vi "UI Flow Rate of Wash Tank.vi"(8 "error in":errorcluster) -> (0 "error out":errorcluster)   [LabVIEW 2019, in "Test.lvlib"]
uses:
  Test.lvlib
  Fluidic Process/SubVI/Fluidic Para.ctl
  <vilib>/Utility/file.llb/Read Delimited Spreadsheet (string).vi
  Controller/Controller.lvlib
  Queues/Queues.lvlib
  Fluidic Process/Fluidic Process.lvlib
panel:
  in  "Stop Process":bool
  out "Remaining Time(s)":dbl
  out "Total Process":string
  out "Current Process":string
  out "Gauge":dbl(knob)=1.2869315802184793e-48 scale=0.0..100.0
  in  "Wash Load R":bool
  in  "Wash Load L":bool
  in  "Back":bool
  # "/"
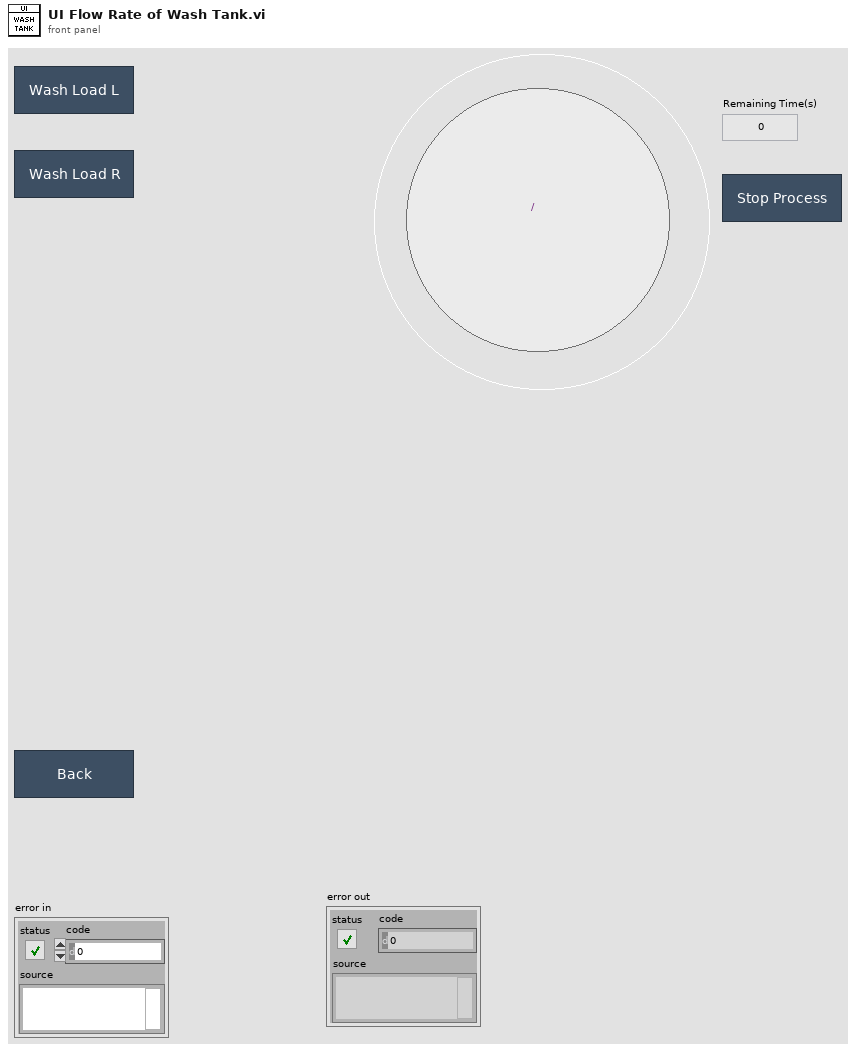
[diagram p1: front panel]
types:
  T1 = enum8{"Enabled", "Disabled", "Disabled and Grayed Out"}
  T2 = typedef "Fluidic Process.lvlib/Fluidic Para.ctl" = cluster{"Read Force Sensor":i32, "Read Regulator":i32, "Read Force Sensor?":bool, "Read Regulator?":bool, "Read Syringe Pump":i32, "Read Syringe Pump?":bool}
  T3 = typedef "Fluidic Process.lvlib/SEQ Data.ctl" = cluster{"Fluidic Process Done?":bool, "Current Process":i32, "Remaining Time":dbl, "Total Process":i32, "Air Sealing":bool, "Force Condition":bool}
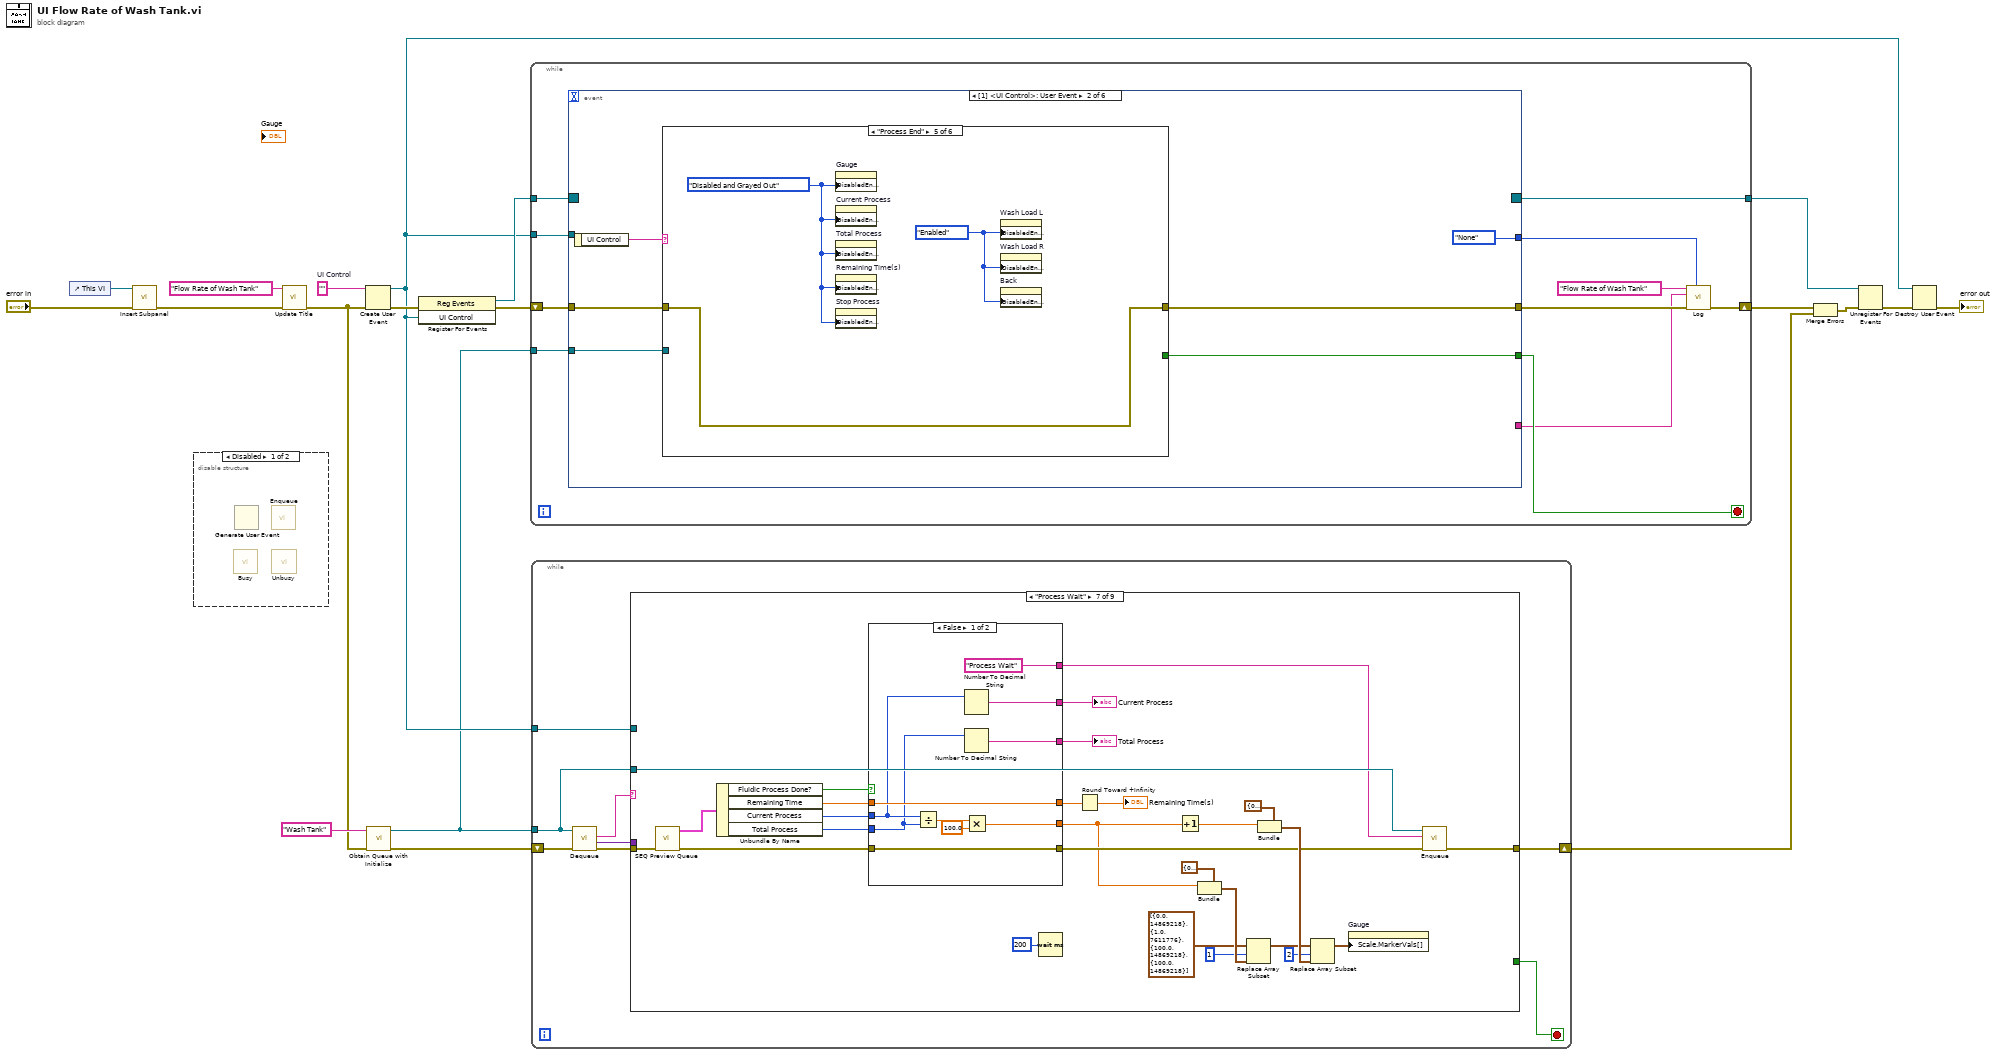
[diagram p0: block diagram]
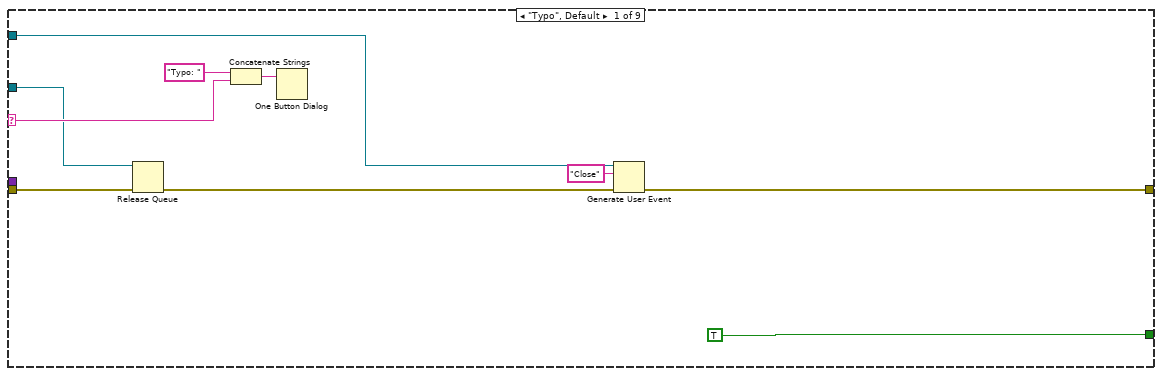
[diagram p3: hidden frame]
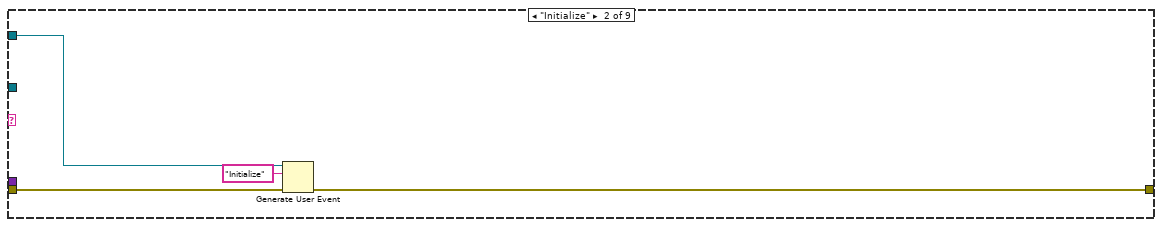
[diagram p4: hidden frame]
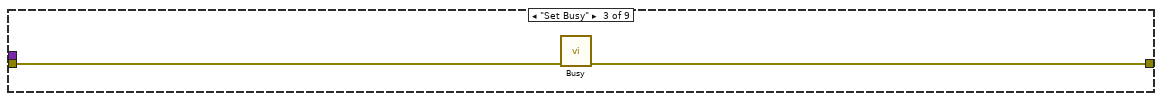
[diagram p5: hidden frame]
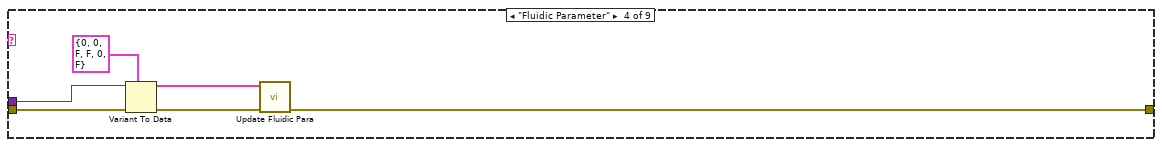
[diagram p6: hidden frame]
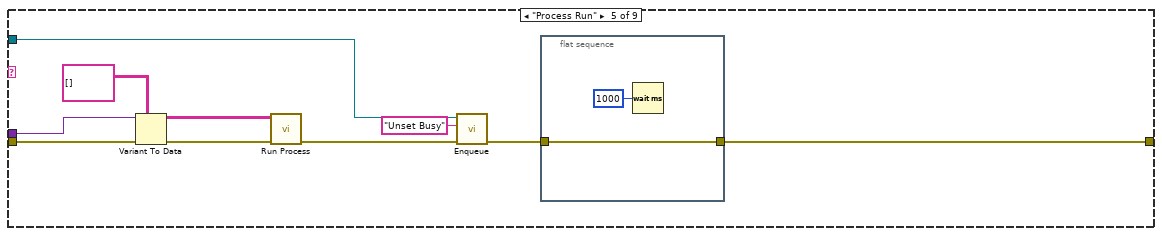
[diagram p7: hidden frame]
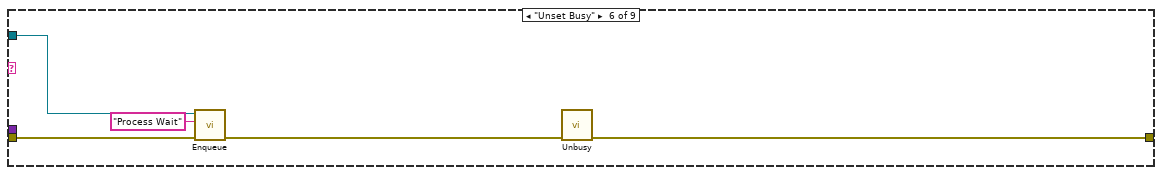
[diagram p8: hidden frame]
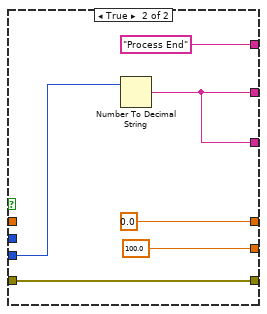
[diagram p9: hidden frame]
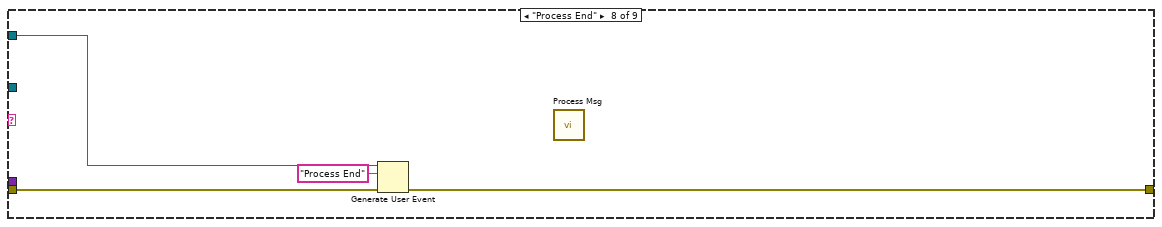
[diagram p10: hidden frame]
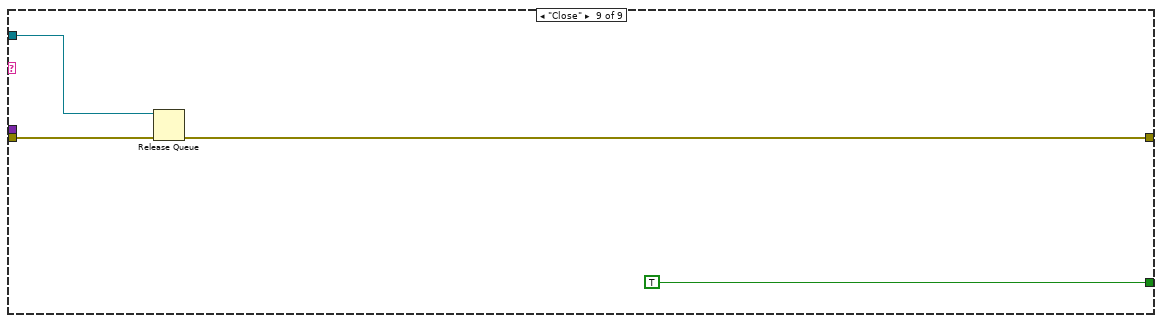
[diagram p11: hidden frame]
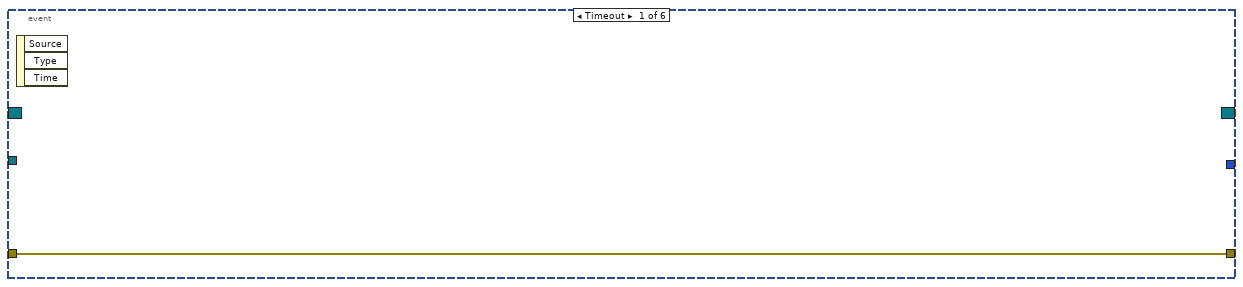
[diagram p12: hidden frame]
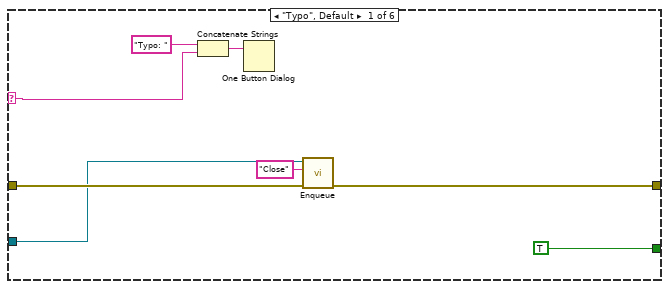
[diagram p13: hidden frame]
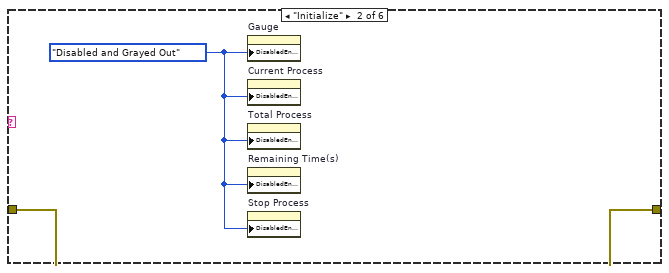
[diagram p14: hidden frame]
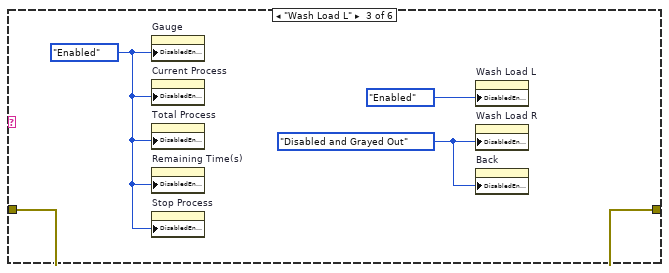
[diagram p15: hidden frame]
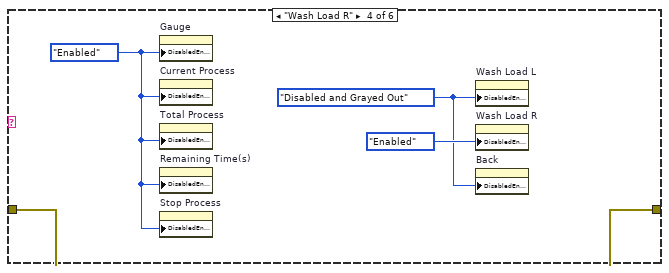
[diagram p16: hidden frame]
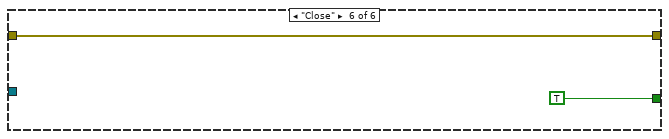
[diagram p17: hidden frame]
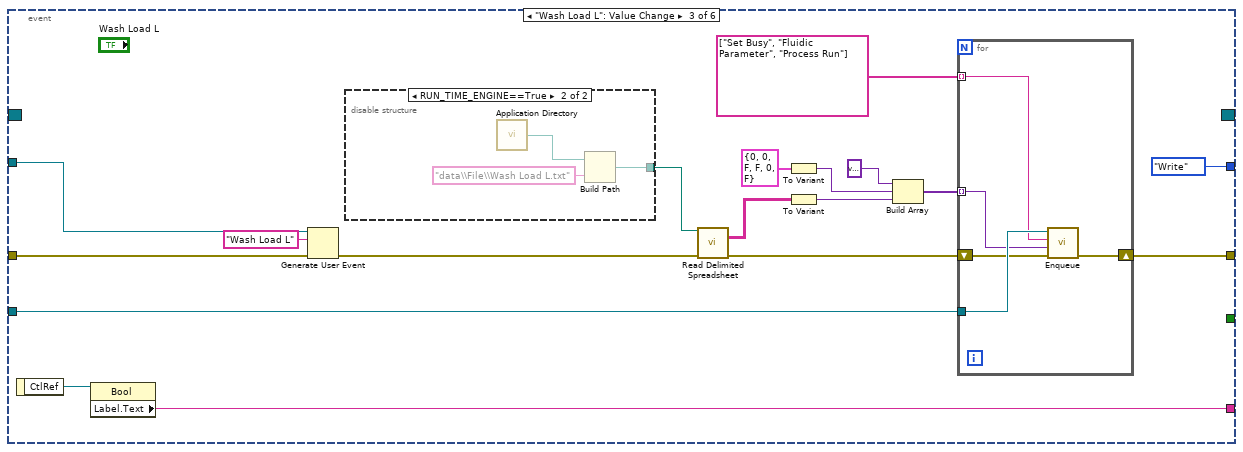
[diagram p18: hidden frame]
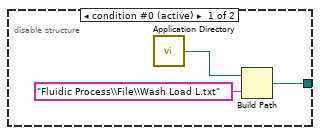
[diagram p19: hidden frame]
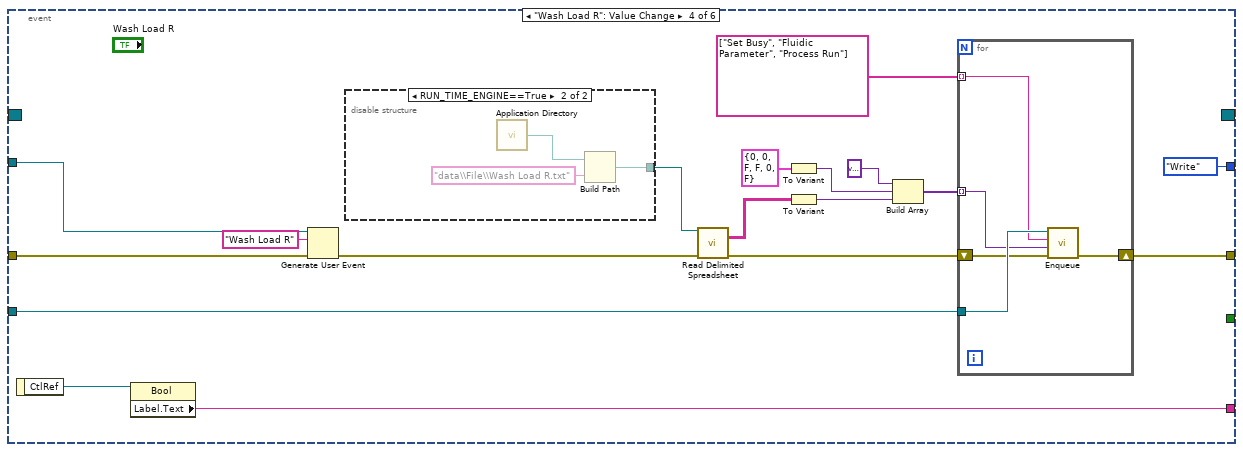
[diagram p20: hidden frame]
diagram:
  w9 = ""  # UI Control
  n1 = control-ref of="This VI"() -> (w8:refnum<vi>)
  n2 = call "Insert Subpanel.vi"("Error In"="error in", "VI Refnum"=w8) -> ("Error Out"=w3:errorcluster)  [unwired: 9 in]
  n3 = disable-structure shown="Disabled" {
    frame Disabled {
      n4 = call "Busy.vi"() -> ()  [unwired: 11 in, 1 out]
      n5 = Generate User Event() -> ()  [unwired: 4 in, 2 out]
      n6 = call "Enqueue.vi"() -> ()  [unwired: 10 in, 2 out]
      n7 = call "Unbusy.vi"() -> ()  [unwired: 11 in, 1 out]
    }
    frame Enabled {
    }
  }
  n8 = call "Update Title.vi"("Error In"=w3, "Title"="Flow Rate of Wash Tank") -> ("Error Out"=w2:errorcluster)  [unwired: 9 in]
  n9 = Create User Event(user event datatype=w9, error in=w2) -> (user event=w7:refnum<user-event>, error out=w18:errorcluster)
  n10 = call "Obtain Queue with Initialize.vi"("Error In"=w2, "Queue Name"="Wash Tank") -> ("Error Out"=w4:errorcluster, "Queue out"=w5:refnum<queue>)  [unwired: 8 in]
  n11 = register-events(error in=w18, w7) -> (reference out=w16:refnum<event-registration>, error out=w17:errorcluster)  [unwired: 1 in]
  n12 = while {
    tunnel: w16 -> [w28]
    tunnel: w5 -> [w27]
    shift-right: [w23] -> w14
    shift-left: w17 -> [w30]
    tunnel: [w26] -> w12
    tunnel: w7 -> [w25]
    stop <- w29 stop-if-true
    n13 = event shown="[1] <UI Control>: User Event" {
      selector: w28 -> [_ _ _ _ _ _]
      dyn-events: [_ _ _ _ _ _] -> w26
      timeout: _ -> [_ _ _ _ _ _]
      tunnel: w30 -> [w31 w37 w67 w96 w123 w127]
      tunnel: [_ w33 _ _ _ TRUE] -> w29
      tunnel: w27 -> [_ w35 w78 w107 _ w129]
      tunnel: [w31 w34 w74 w103 w122 w130] -> w24
      tunnel: w25 -> [_ _ w65 w94 _ _]
      tunnel: [_ enum16{"None", "Write"}."None" ("Action") enum16{"None", "Write"}."Write" ("Action") enum16{"None", "Write"}."Write" ("Action") enum16{"None", "Write"}."Write" ("Action") enum16{"None", "Write"}."Write" ("Action")] -> w21
      tunnel: [_ _ w61 w90 w120 w125] -> w20
      event Timeout {
        n14 = event-data() -> ()  [unwired: 1 in, 3 out]
      }
      event User Event {
        n15 = event-data() -> ("UI Control"=w36:string)  [unwired: 1 in]
        n16 = case shown="\"Process End\"" w36 {
          selector: w36 -> [w40 _ _ _ _ _]
          tunnel: w37 -> [w45 w47 w51 w55 w58 w60]
          tunnel: w35 -> [w44 _ _ _ _ _]
          tunnel: [w39 w47 w51 w55 w58 w60] -> w34
          tunnel: [TRUE _ _ _ _ TRUE] -> w33
          frame "Typo", Default {
            n17 = Concatenate Strings("Typo: " ("string"), w40) -> (w41:string)
            n18 = One Button Dialog(message=w41) -> ()  [unwired: 1 in, 1 out]
            n19 = call "Enqueue.vi"("Error In"=w45, "State"="Close", "Queue in"=w44) -> ("Error Out"=w39:errorcluster)  [unwired: 7 in, 1 out]
          }
          frame "Initialize" {
            w46 = T1."Disabled and Grayed Out" ("Disabled")
            n20 = property on="Gauge" class="Knob (strict)"("DisabledEnum"=w46) -> ()  [unwired: 2 in, 2 out]
            n21 = property on="Current Process" class="Str"("DisabledEnum"=w46) -> ()  [unwired: 2 in, 2 out]
            n22 = property on="Total Process" class="Str"("DisabledEnum"=w46) -> ()  [unwired: 2 in, 2 out]
            n23 = property on="Remaining Time(s)" class="DigNum (strict)"("DisabledEnum"=w46) -> ()  [unwired: 2 in, 2 out]
            n24 = property on="Stop Process" class="Bool"("DisabledEnum"=w46) -> ()  [unwired: 2 in, 2 out]
          }
          frame "Wash Load L" {
            w49 = T1."Enabled" ("Disabled")
            w48 = T1."Disabled and Grayed Out" ("Disabled")
            n25 = property on="Gauge" class="Knob (strict)"("DisabledEnum"=w49) -> ()  [unwired: 2 in, 2 out]
            n26 = property on="Current Process" class="Str"("DisabledEnum"=w49) -> ()  [unwired: 2 in, 2 out]
            n27 = property on="Total Process" class="Str"("DisabledEnum"=w49) -> ()  [unwired: 2 in, 2 out]
            n28 = property on="Remaining Time(s)" class="DigNum (strict)"("DisabledEnum"=w49) -> ()  [unwired: 2 in, 2 out]
            n29 = property on="Stop Process" class="Bool"("DisabledEnum"=w49) -> ()  [unwired: 2 in, 2 out]
            n30 = property on="Wash Load L" class="Bool"("DisabledEnum"=T1."Enabled" ("Disabled")) -> ()  [unwired: 2 in, 2 out]
            n31 = property on="Wash Load R" class="Bool"("DisabledEnum"=w48) -> ()  [unwired: 2 in, 2 out]
            n32 = property on="Back" class="Bool"("DisabledEnum"=w48) -> ()  [unwired: 2 in, 2 out]
          }
          frame "Wash Load R" {
            w53 = T1."Enabled" ("Disabled")
            w52 = T1."Disabled and Grayed Out" ("Disabled")
            n33 = property on="Gauge" class="Knob (strict)"("DisabledEnum"=w53) -> ()  [unwired: 2 in, 2 out]
            n34 = property on="Current Process" class="Str"("DisabledEnum"=w53) -> ()  [unwired: 2 in, 2 out]
            n35 = property on="Total Process" class="Str"("DisabledEnum"=w53) -> ()  [unwired: 2 in, 2 out]
            n36 = property on="Remaining Time(s)" class="DigNum (strict)"("DisabledEnum"=w53) -> ()  [unwired: 2 in, 2 out]
            n37 = property on="Stop Process" class="Bool"("DisabledEnum"=w53) -> ()  [unwired: 2 in, 2 out]
            n38 = property on="Wash Load L" class="Bool"("DisabledEnum"=w52) -> ()  [unwired: 2 in, 2 out]
            n39 = property on="Wash Load R" class="Bool"("DisabledEnum"=T1."Enabled" ("Disabled")) -> ()  [unwired: 2 in, 2 out]
            n40 = property on="Back" class="Bool"("DisabledEnum"=w52) -> ()  [unwired: 2 in, 2 out]
          }
          frame "Process End" {
            w57 = T1."Disabled and Grayed Out" ("Disabled")
            w56 = T1."Enabled" ("Disabled")
            n41 = property on="Gauge" class="Knob (strict)"("DisabledEnum"=w57) -> ()  [unwired: 2 in, 2 out]
            n42 = property on="Current Process" class="Str"("DisabledEnum"=w57) -> ()  [unwired: 2 in, 2 out]
            n43 = property on="Total Process" class="Str"("DisabledEnum"=w57) -> ()  [unwired: 2 in, 2 out]
            n44 = property on="Remaining Time(s)" class="DigNum (strict)"("DisabledEnum"=w57) -> ()  [unwired: 2 in, 2 out]
            n45 = property on="Stop Process" class="Bool"("DisabledEnum"=w57) -> ()  [unwired: 2 in, 2 out]
            n46 = property on="Wash Load L" class="Bool"("DisabledEnum"=w56) -> ()  [unwired: 2 in, 2 out]
            n47 = property on="Wash Load R" class="Bool"("DisabledEnum"=w56) -> ()  [unwired: 2 in, 2 out]
            n48 = property on="Back" class="Bool"("DisabledEnum"=w56) -> ()  [unwired: 2 in, 2 out]
          }
          frame "Close" {
          }
        }
      }
      event "Wash Load L": Value Change {
        n49 = event-data() -> ("CtlRef"=w62:refnum<vi>)  [unwired: 1 in]
        n50 = property class="Bool"(reference=w62) -> ("Label.Text"=w61:string)  [unwired: 1 in, 2 out]
        n51 = Generate User Event(user event=w65, event data cluster="Wash Load L" ("event data"), error in=w67) -> (error out=w66:errorcluster)  [unwired: 1 in, 1 out]
        n52 = disable-structure shown="RUN_TIME_ENGINE==True" {
          disable-tunnel: [w79 w82] -> w76
          frame condition #0 (active) {
            n53 = call <vilib>:"Application Directory.vi"() -> ("Application Directory"=w81:path)
            n54 = Build Path(base path=w81, name or relative path="Fluidic Process\\File\\Wash Load L.txt") -> (appended path=w79:path)
          }
          frame condition #1 {
            n55 = call <vilib>:"Application Directory.vi"() -> ("Application Directory"=w84:path)
            n56 = Build Path(base path=w84, name or relative path="data\\File\\Wash Load L.txt") -> (appended path=w82:path)
          }
        }
        n57 = call-poly <vilib>:"Read Delimited Spreadsheet.vi"("file path (dialog if empty)"=w76, "error in (no error)"=w66) -> ("all rows"=w75:string[][], "error out"=w77:errorcluster)  [unwired: 8 in, 4 out]
        n58 = To Variant(anything=T2 {"Read Force Sensor"=0, "Read Regulator"=0, "Read Force Sensor?"=FALSE, "Read Regulator?"=FALSE, "Read Syringe Pump"=0, "Read Syringe Pump?"=FALSE} ("Cluster")) -> (Variant=w70:variant)
        n59 = To Variant(anything=w75) -> (Variant=w72:variant)
        n60 = Build Array(variant, w70, w72) -> (w69:variant[])
        n61 = for {
          tunnel: w78 -> [w89]
          shift-right: [w87] -> w74
          shift-left: w77 -> [w88]
          tunnel: string[] ["Set Busy", "Fluidic Parameter", "Process Run"] -> [w86] mode=indexing
          tunnel: w69 -> [w85] mode=indexing
          n62 = call "Enqueue.vi"("Error In"=w88, "Data"=w85, "State"=w86, "Queue in"=w89) -> ("Error Out"=w87:errorcluster)  [unwired: 6 in, 1 out]
        }
      }
      event "Wash Load R": Value Change {
        n63 = event-data() -> ("CtlRef"=w91:refnum<vi>)  [unwired: 1 in]
        n64 = property class="Bool"(reference=w91) -> ("Label.Text"=w90:string)  [unwired: 1 in, 2 out]
        n65 = Generate User Event(user event=w94, event data cluster="Wash Load R" ("event data"), error in=w96) -> (error out=w95:errorcluster)  [unwired: 1 in, 1 out]
        n66 = disable-structure shown="RUN_TIME_ENGINE==True" {
          disable-tunnel: [w108 w111] -> w105
          frame condition #0 (active) {
            n67 = call <vilib>:"Application Directory.vi"() -> ("Application Directory"=w110:path)
            n68 = Build Path(base path=w110, name or relative path="Fluidic Process\\File\\Wash Load R.txt") -> (appended path=w108:path)
          }
          frame condition #1 {
            n69 = call <vilib>:"Application Directory.vi"() -> ("Application Directory"=w113:path)
            n70 = Build Path(base path=w113, name or relative path="data\\File\\Wash Load R.txt") -> (appended path=w111:path)
          }
        }
        n71 = call-poly <vilib>:"Read Delimited Spreadsheet.vi"("file path (dialog if empty)"=w105, "error in (no error)"=w95) -> ("all rows"=w104:string[][], "error out"=w106:errorcluster)  [unwired: 8 in, 4 out]
        n72 = To Variant(anything=T2 {"Read Force Sensor"=0, "Read Regulator"=0, "Read Force Sensor?"=FALSE, "Read Regulator?"=FALSE, "Read Syringe Pump"=0, "Read Syringe Pump?"=FALSE} ("Cluster")) -> (Variant=w99:variant)
        n73 = To Variant(anything=w104) -> (Variant=w101:variant)
        n74 = Build Array(variant, w99, w101) -> (w98:variant[])
        n75 = for {
          tunnel: w107 -> [w118]
          shift-right: [w116] -> w103
          shift-left: w106 -> [w117]
          tunnel: string[] ["Set Busy", "Fluidic Parameter", "Process Run"] -> [w115] mode=indexing
          tunnel: w98 -> [w114] mode=indexing
          n76 = call "Enqueue.vi"("Error In"=w117, "Data"=w114, "State"=w115, "Queue in"=w118) -> ("Error Out"=w116:errorcluster)  [unwired: 6 in, 1 out]
        }
      }
      event "Stop Process": Value Change {
        n77 = event-data() -> ("CtlRef"=w121:refnum<vi>)  [unwired: 1 in]
        n78 = property class="Bool"(reference=w121) -> ("Label.Text"=w120:string)  [unwired: 1 in, 2 out]
        n79 = call "Stop Process.vi"("Error In"=w123) -> ("Error Out"=w122:errorcluster)  [unwired: 10 in]
      }
      event "Back": Value Change {
        n80 = event-data() -> ("CtlRef"=w126:refnum<vi>)  [unwired: 1 in]
        n81 = property class="Bool"(reference=w126) -> ("Label.Text"=w125:string)  [unwired: 1 in, 2 out]
        n82 = call "Enqueue.vi"("Error In"=w127, "State"="Close", "Queue in"=w129) -> ("Error Out"=w130:errorcluster)  [unwired: 7 in, 1 out]
      }
    }
    n83 = call "Log.vi"("Action"=w21, "error in"=w24, "State"=w20, "Page Name"="Flow Rate of Wash Tank") -> ("error out"=w23:errorcluster)  [unwired: 7 in]
  }
  n84 = while {
    tunnel: w5 -> [w136]
    shift-right: [w134] -> w13
    shift-left: w4 -> [w139]
    tunnel: w7 -> [w133]
    stop <- w132 stop-if-true
    n85 = call "Dequeue.vi"("Error In"=w139, "Queue in"=w136) -> ("Error Out"=w135:errorcluster, "Data"=w137:variant, "State"=w138:string)  [unwired: 6 in, 1 out]
    n86 = case shown="\"Process Wait\"" w138 {
      selector: w138 -> [w147 _ _ _ _ _ _ _ _]
      tunnel: w137 -> [_ _ _ w160 w170 _ _ _ _]
      tunnel: w136 -> [w140 _ _ _ w165 w177 w183 _ w227]
      tunnel: w135 -> [w142 w153 w155 w161 w171 w178 w205 w225 w229]
      tunnel: [TRUE _ _ _ _ _ _ _ TRUE] -> w132
      tunnel: [w145 w152 w154 w156 w162 w174 w189 w224 w228] -> w134
      tunnel: w133 -> [w144 w151 _ _ _ _ _ w223 _]
      frame "Typo", Default {
        n87 = Release Queue(queue=w140, error in (no error)=w142) -> (error out=w141:errorcluster)  [unwired: 1 in, 2 out]
        n88 = Concatenate Strings("Typo: " ("string"), w147) -> (w149:string)
        n89 = One Button Dialog(message=w149) -> ()  [unwired: 1 in, 1 out]
        n90 = Generate User Event(user event=w144, event data cluster="Close" ("event data"), error in=w141) -> (error out=w145:errorcluster)  [unwired: 1 in, 1 out]
      }
      frame "Initialize" {
        n91 = Generate User Event(user event=w151, event data cluster="Initialize" ("event data"), error in=w153) -> (error out=w152:errorcluster)  [unwired: 1 in, 1 out]
      }
      frame "Set Busy" {
        n92 = call "Busy.vi"("Error In"=w155) -> ("Error Out"=w154:errorcluster)  [unwired: 10 in]
      }
      frame "Fluidic Parameter" {
        n93 = Variant To Data(error in=w161, type=T2 {"Read Force Sensor"=0, "Read Regulator"=0, "Read Force Sensor?"=FALSE, "Read Regulator?"=FALSE, "Read Syringe Pump"=0, "Read Syringe Pump?"=FALSE} ("Cluster"), Variant=w160) -> (data=w157:T2, error out=w158:errorcluster)
        n94 = call "Update Fluidic Para.vi"("Error In"=w158, "Fluidic Para"=w157) -> ("Error Out"=w156:errorcluster)  [unwired: 9 in]
      }
      frame "Process Run" {
        n95 = Variant To Data(error in=w171, type=string[][] [] ("all rows"), Variant=w170) -> (data=w167:string[][], error out=w168:errorcluster)
        n96 = call "Run Process.vi"("Error In"=w168, "Fluidic Process in"=w167) -> ("Error Out"=w166:errorcluster)  [unwired: 9 in]
        n97 = call "Enqueue.vi"("Error In"=w166, "State"="Unset Busy", "Queue in"=w165) -> ("Error Out"=w163:errorcluster)  [unwired: 7 in, 1 out]
        n98 = flat-sequence {
          tunnel: w163 -> [w173]
          tunnel: [w173] -> w162
          frame #0 {
            n99 = Wait (ms)(milliseconds to wait=u32 1000) -> ()  [unwired: 1 out]
          }
        }
      }
      frame "Unset Busy" {
        n100 = call "Enqueue.vi"("Error In"=w178, "State"="Process Wait", "Queue in"=w177) -> ("Error Out"=w175:errorcluster)  [unwired: 7 in, 1 out]
        n101 = call "Unbusy.vi"("Error In"=w175) -> ("Error Out"=w174:errorcluster)  [unwired: 10 in]
      }
      frame "Process Wait" {
        n102 = call "SEQ Preview Queue.vi"("error in"=w205) -> ("error out"=w202:errorcluster, "SEQ Data"=w204:T3)  [unwired: 9 in]
        n103 = Unbundle By Name(w204) -> ("Fluidic Process Done?"=w203:bool, "Remaining Time"=w188:dbl, "Current Process"=w187:i32, "Total Process"=w186:i32)
        n104 = case shown="False" w203 {
          tunnel: w202 -> [w213 w221]
          tunnel: [w213 w221] -> w190
          tunnel: w188 -> [w212 _]
          tunnel: w187 -> [w210 _]
          tunnel: w186 -> [w209 w220]
          tunnel: [w212 0.0 ("Remaining Time")] -> w184
          tunnel: [w211 100.0] -> w185
          tunnel: [w208 w219] -> w182
          tunnel: [w207 w219] -> w181
          tunnel: ["Process Wait" "Process End"] -> w180
          frame False {
            n105 = Divide(x=w210, y=w209) -> (x/y=w215:dbl)
            n106 = Number To Decimal String(number=w210) -> (decimal integer string=w208:string)  [unwired: 1 in]
            n107 = Number To Decimal String(number=w209) -> (decimal integer string=w207:string)  [unwired: 1 in]
            n108 = Multiply(x=w215, y=100.0) -> (x*y=w211:dbl)
          }
          frame True {
            n109 = Number To Decimal String(number=w220) -> (decimal integer string=w219:string)  [unwired: 1 in]
          }
        }
        "Total Process" <- w181
        "Current Process" <- w182
        n110 = Wait (ms)(milliseconds to wait=u32 200) -> ()  [unwired: 1 out]
        n111 = Round Toward +Infinity(x=w184) -> (ceil(x): smallest int >= x=→"Remaining Time(s)":dbl)
        n112 = Increment(x=w185) -> (x+1=w198:dbl)
        n113 = Bundle(cluster=cluster{dbl, i32} {0.0, 7611776}, w185) -> (w197:cluster{dbl, i32})  [unwired: 1 in]
        n114 = Replace Array Subset(array=cluster{dbl, u32}[] [{0.0, 14869218}, {1.0, 7611776}, {100.0, 14869218}, {100.0, 14869218}] ("Scale.Marker Values[]"), new element=w197, index=1) -> (w199:cluster{dbl, u32}[])
        n115 = Bundle(cluster=cluster{dbl, i32} {0.0, 14869218}, w198) -> (w200:cluster{dbl, i32})  [unwired: 1 in]
        n116 = Replace Array Subset(array=w199, new element=w200, index=2) -> (w201:cluster{dbl, u32}[])
        n117 = property on="Gauge" class="Knob (strict)"("Scale.MarkerVals[]"=w201) -> ()  [unwired: 2 in, 2 out]
        n118 = call "Enqueue.vi"("Error In"=w190, "State"=w180, "Queue in"=w183) -> ("Error Out"=w189:errorcluster)  [unwired: 7 in, 1 out]
      }
      frame "Process End" {
        n119 = Generate User Event(user event=w223, event data cluster="Process End" ("event data"), error in=w225) -> (error out=w224:errorcluster)  [unwired: 1 in, 1 out]
        n120 = call "Process Msg"() -> ()  [unwired: 10 in, 2 out]
      }
      frame "Close" {
        n121 = Release Queue(queue=w227, error in (no error)=w229) -> (error out=w228:errorcluster)  [unwired: 1 in, 2 out]
      }
    }
  }
  n122 = Merge Errors(w14, w13) -> (w11:errorcluster)
  n123 = Unregister For Events(event registration refnum=w12, error in=w11) -> (error out=w10:errorcluster)
  n124 = Destroy User Event(user event=w7, error in=w10) -> (error out=→"error out":errorcluster)
